vi "1WIRE_Write_1_bit_9402.vi"(8 "error in":errorcluster) -> (0 "error out":errorcluster)   [LabVIEW 2012]
doc: "This VI is created by Vincent Claes for FPDA-1 more information on http://pwo.fpga.be\n\nvincent.claes@xios.be\nclaesvincent@gmail.com\n\nhttp://www.linkedin.com/in/vincentclaes"
uses:
  <vilib>/rvi/eio/common/nirviEmuTemplateMethod_errors.vi
  <vilib>/eio/EIOMethodNode/EIOMethodNode.xnode
  <vilib>/eio/EIONode/EIONode.xnode
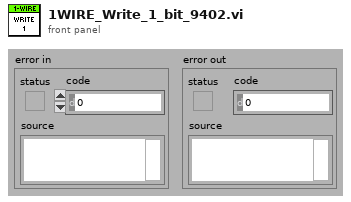
[diagram p1: front panel]
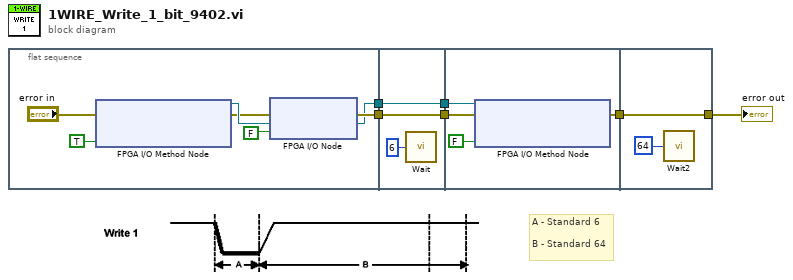
[diagram p0: block diagram]
diagram:
  # "A - Standard 6\n\nB - Standard 64"
  n1 = flat-sequence {
    tunnel: [w8] -> w5
    tunnel: [w7] -> w2
    tunnel: w5 -> [w16]
    tunnel: [w16] -> w4
    tunnel: w2 -> [w15]
    tunnel: [w15] -> w1
    tunnel: w4 -> [w18]
    tunnel: [w19] -> w3
    tunnel: w1 -> [w17]
    tunnel: [w21] -> w6
    tunnel: w3 -> [w21]
    frame #0 {
      n2 = xnode "FPGA I/O Method Node"("error in"="error in", "Enable"=TRUE) -> ("error out"=w10:errorcluster, "FPGA I/O Out"=w12:refnum<k21>)  [unwired: 1 in]
      n3 = xnode "FPGA I/O Node"("error in"=w10, "I/O Item"=FALSE ("FX2_IO1_J1_0"), "FPGA I/O In"=w12) -> ("error out"=w8:errorcluster, "FPGA I/O Out"=w7:refnum<k21>)
    }
    frame #1 {
      n4 = call "Wait"("Count(uSec)"=u32 6) -> ()  [unwired: 1 out]
    }
    frame #2 {
      n5 = xnode "FPGA I/O Method Node"("error in"=w18, "FPGA I/O In"=w17, "Enable"=FALSE) -> ("error out"=w19:errorcluster)  [unwired: 1 out]
    }
    frame #3 {
      n6 = call "Wait2"("Count(uSec)"=u32 64) -> ()  [unwired: 1 out]
    }
  }
  "error out" <- w6
